vi "Clear errors.vi"(8 "error in":errorcluster) -> (0 "error out":errorcluster, 1 "Clear?":bool, 2 "code":i32)   [LabVIEW 2014, in "Generic Instrument.lvlib" / "Generic Instrument.lvclass"]
uses:
  Generic Instrument.lvclass
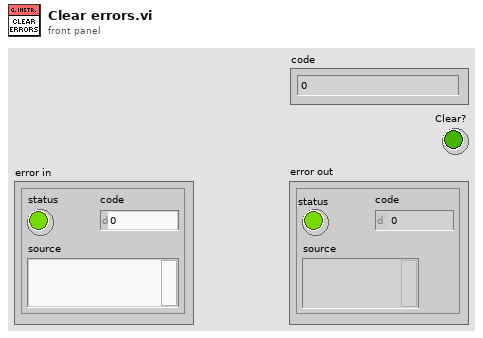
[diagram p1: front panel]
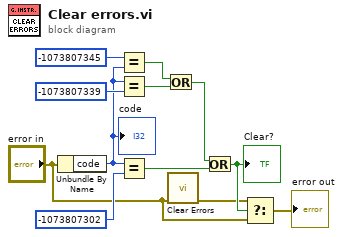
[diagram p0: block diagram]
diagram:
  n1 = Unbundle By Name("error in") -> ("code"=w3:i32)
  "code" <- w3
  n2 = Equal?(x=-1073807345, y=w3) -> (x = y?=w11:bool)
  n3 = Equal?(x=w3, y=-1073807339) -> (x = y?=w6:bool)
  n4 = Equal?(x=w3, y=-1073807302) -> (x = y?=w4:bool)
  n5 = Or(x=w11, y=w6) -> (x .or. y?=w10:bool)
  n6 = call <vilib>:"Clear Errors.vi"("error in (no error)"="error in") -> ("error out"=w8:errorcluster)  [unwired: 5 in, 1 out]
  n7 = Or(x=w10, y=w4) -> (x .or. y?=w9:bool)
  "Clear?" <- w9
  n8 = Select(t=w8, s=w9, f="error in") -> (s? t:f=→"error out":errorcluster)
